vi "MonitorCommunications.vi"() -> ()   [LabVIEW 2009]
panel:
  in  "stop":bool
  out "Messages":string="?SEL\r\n0\r\n\r>?SEL\r\n0\r\n\r>?SEL\r\n0\r\n\r>SEL 5\r\n>MVT -500\r\n>?POS\r\n121077\r\n\r>?POS\r\n121035\r\n\r>?POS\r\n120993\r\n\r>?POS\r\n120949\r\n\r>?POS\r\n120907\r\n\r>?POS\r\n120866\r\n\r>?POS\r\n120824\r\n\r>?POS\r\n120782\r\n\r>?POS\r\n120738\r\n\r>?POS\r\n120696\r\n\r>?POS\r\n120653\r\n\r>?POS\r\n121115\r\n\r>?POS\r\n120615\r\n\r>?POS\r\n120615\r\n\r>?POS\r\n120615\r\n\r>?POS\r\n120615\r\n\r>?POS\r\n120615\r\n\r>?POS\r\n120615\r\n\r>?POS\r\n120615\r\n\r>?POS\r\n120615\r\n\r>?POS\r\n120615\r\n\r>MVT 500\r\n>?POS\r\n120653\r\n\r>?POS\r\n120696\r\n\r>?POS\r\n120739\r\n\r>?POS\r\n120781\r\n\r>?POS\r\n120823\r\n\r>?POS\r\n120865\r\n\r>?POS\r\n120908\r\n\r>?POS\r\n120949\r\n\r>?POS\r\n120991\r\n\r>?POS\r\n121033\r\n\r>?POS\r\n121077\r\n\r>?POS\r\n120615\r\n\r>?POS\r\n121115\r\n\r>?POS\r\n121115\r\n\r>?POS\r\n121115\r\n\r>?POS\r\n121115\r\n\r>?POS\r\n121115\r\n\r>?POS\r\n121115\r\n\r>?SEL\r\n5\r\n\r>SEL 0\r\n>"
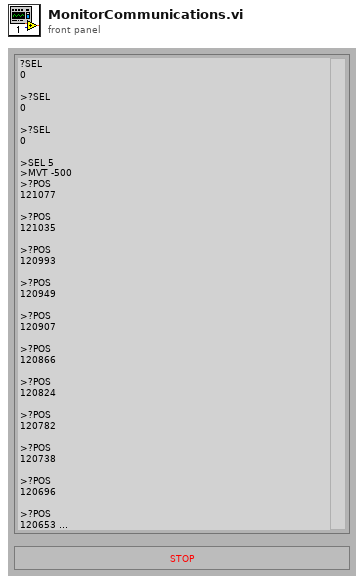
[diagram p1: front panel]
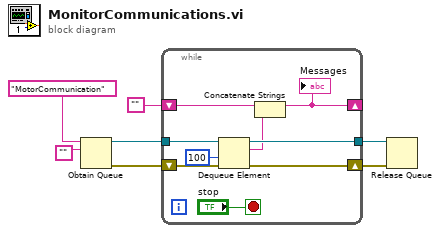
[diagram p0: block diagram]
diagram:
  n1 = Obtain Queue(name (unnamed)="MotorCommunication", element data type="") -> (queue out=w4:refnum<queue>, error out=w5:errorcluster)  [unwired: 3 in, 1 out]
  n2 = while {
    shift-right: [w14] -> w1
    shift-left: w5 -> [w15]
    tunnel: w4 -> [w13]
    tunnel: [w11] -> w3
    shift-right: [w8] -> _
    shift-left: "" -> [w10]
    stop <- "stop" stop-if-true
    n3 = Dequeue Element(queue=w13, timeout in ms (-1)=100 ("timeout en ms (-1)"), error in (no error)=w15) -> (queue out=w11:refnum<queue>, element=w9:string, error out=w14:errorcluster)  [unwired: 1 out]
    n4 = Concatenate Strings(w10, w9) -> (w8:string)
    "Messages" <- w8
  }
  n5 = Release Queue(queue=w3, error in (no error)=w1) -> ()  [unwired: 4 out]
